vi "CALC_FILT_GATE_TIME_SHAP.vi"(0 "VISA IN":refnum<visa-resource-name>, 1 "FilterShape":string(combo), 5 "error in":errorcluster, 7 "Channel":i32) -> (14 "VISA Out":refnum<visa-resource-name>, 19 "error out":errorcluster)   [LabVIEW 2018, in "PNA-X.lvlib"]
doc: "CALCulate<cnum>:FILTer[:GATE]:TIME:SHAPe <char> \n(Read-Write) Sets the gating filter shape when in time domain. \nSee Critical Note \nParameters \n<cnum> Channel number of the measurement. There must be a selected measurement \non that channel. If unspecified, <cnum> is set to 1. \n<char> Choose from \nMAXimum - the widest gate filter available \nWIDE - \nNORMal - \nMINimum - the narrowest gate filter available \nExamples CALC:FILT:GATE:TIME:SHAP MAX \ncalculate2:filter:time:shape normal \nQuery Syntax CALCulate<cnum>:FILTer[:GATE]:TIME:SHAPe? \nReturn Type Character \nDefault NORMal \n1508"
uses:
  PNA-X.lvlib
panel:
  # "MAXimum - the widest gate filter available\nWIDE -\nNORMal -\nMINimum"
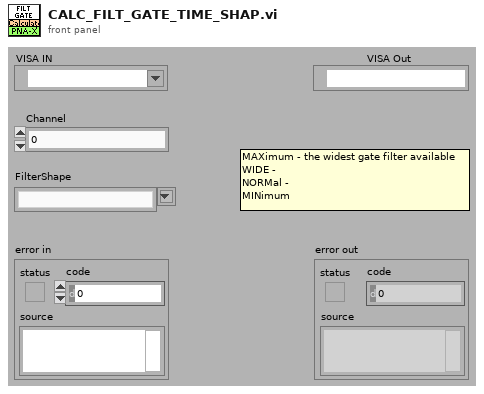
[diagram p1: front panel]
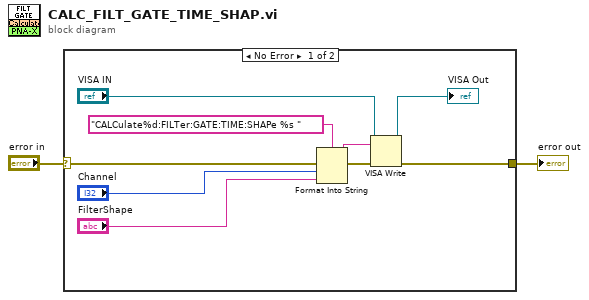
[diagram p0: block diagram]
diagram:
  n1 = case shown="No Error" "error in" {
    selector: "error in" -> [w11 w12]
    tunnel: [w6 w12] -> w1
    frame No Error {
      n2 = Format Into String(format string="CALCulate%d:FILTer:GATE:TIME:SHAPe %s " ("Cmdline"), error in=w11, "Channel", "FilterShape") -> (resulting string=w9:string, error out=w10:errorcluster)  [unwired: 1 in]
      n3 = VISA Write(VISA resource name="VISA IN", write buffer=w9, error in (no error)=w10) -> (VISA resource name out=→"VISA Out":refnum<visa-resource-name>, error out=w6:errorcluster)  [unwired: 1 out]
    }
    frame Error {
    }
  }
  "error out" <- w1
